vi "UnFlatten Driver Parameters.vi"(4 "error in (no error)":errorcluster, 7 "Flattened Driver Parameters with Version (\"\")":string) -> (0 "error out":errorcluster, 2 "Driver Version":string, 3 "Flat Driver Parameters":string)   [LabVIEW 2011]
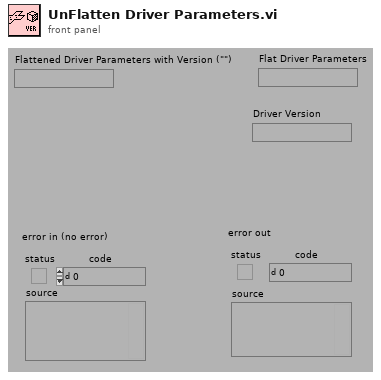
[diagram p1: front panel]
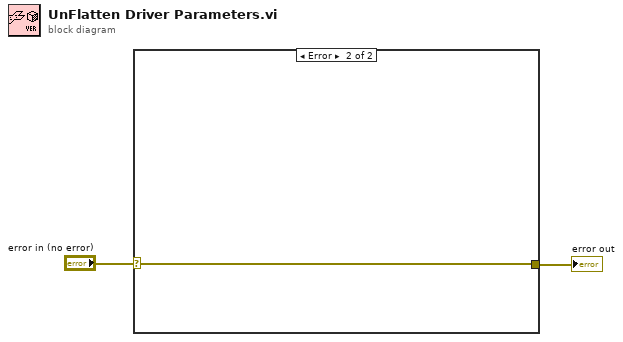
[diagram p0: block diagram]
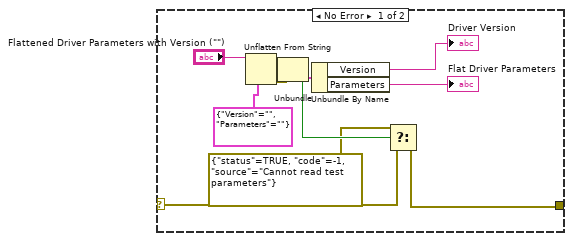
[diagram p2: hidden frame]
diagram:
  n1 = case shown="Error" "error in (no error)" {
    selector: "error in (no error)" -> [w4 w13]
    tunnel: [w5 w13] -> w2
    frame No Error {
      n2 = Unflatten From String(type=cluster{"Version":string, "Parameters":string} {"Version"="", "Parameters"=""}, binary string="Flattened Driver Parameters with Version (\"\")") -> (value=w10:cluster{"Version":string, "Parameters":string}, error out=w3:errorcluster)  [unwired: 1 in, 3 out]
      n3 = Unbundle(w3) -> ("status"=w7:bool)  [unwired: 2 out]
      n4 = Unbundle By Name(w10) -> ("Version"=→"Driver Version":string, "Parameters"=→"Flat Driver Parameters":string)
      n5 = Select(t=errorcluster {"status"=TRUE, "code"=-1, "source"="Cannot read test parameters"}, s=w7, f=w4) -> (s? t:f=w5:errorcluster)
    }
    frame Error {
    }
  }
  "error out" <- w2
